vi "datascope.from_json.vi"(8 "error in":errorcluster, 10 "json":string) -> (0 "error out":errorcluster, 2 "data scope":T1)   [LabVIEW 2020, in "dataScopes.lvlib"]
uses:
  dataScopes.lvlib
  data_scope.ctl
  properties/properties.lvclass
  data_source.ctl
  type.ctl
  offset.ctl
  67163aca-3a6b-4dd5-86ca-74d13fcabb29.vi
  ab9a869c-e1cd-4f12-85c3-02f872140d20.vi
  <vilib>/JDP Science/JSONtext/Find Item.vi
  <vilib>/JDP Science/JSONtext/String Subset.vi
  <vilib>/JDP Science/JSONtext/Offset/Find Object Item Locations by Names.vi
  <vilib>/JDP Science/JSONtext/support/Quote and Escape JSON string.vi
  <vilib>/JDP Science/JSONtext/Next JSON Value.vi
  <vilib>/JDP Science/JSONtext/Parsing/Advance past whitespace.vi
  <vilib>/JDP Science/JSONtext/support/Commas Needed.vi
  <vilib>/JDP Science/JSONtext/Parsing/Advance past whitespace and comma.vi
  <vilib>/JDP Science/JSONtext/Parsing/Advance past next JSON Value (inlined COPY).vi
  <vilib>/JDP Science/JSONtext/Parsing/Advance past Item Name.vi
  <vilib>/JDP Science/JSONtext/support/quote and escape json string 2.vi
  <vilib>/JDP Science/JSONtext/Parsing/Advance past Line Ending.vi
  <vilib>/JDP Science/JSONtext/Parsing/Advance past String.vi
  <vilib>/JDP Science/JSONtext/Parsing/Advance past Number.vi
  <vilib>/JDP Science/JSONtext/Parsing/Parse Full Path or Item Name.vi
  <vilib>/JDP Science/JSONtext/Parsing/Advance past Array.vi
  <vilib>/JDP Science/JSONtext/Parsing/Advance past Object.vi
  <vilib>/JDP Science/JSONtext/support/Error Cluster From Code.vi
  <vilib>/JDP Science/JSONtext/Offset/Find Item Locations by Path.vi
  <vilib>/JDP Science/JSONtext/Parsing/Parsing Error.vi
  <vilib>/JDP Science/JSONtext/JSON text to Variant.vi
  <vilib>/JDP Science/JSONtext/LVClass Serializer/JSONtext LVClass Serializer.lvclass
  <vilib>/JDP Science/JSONtext/JSONtext.lvlib
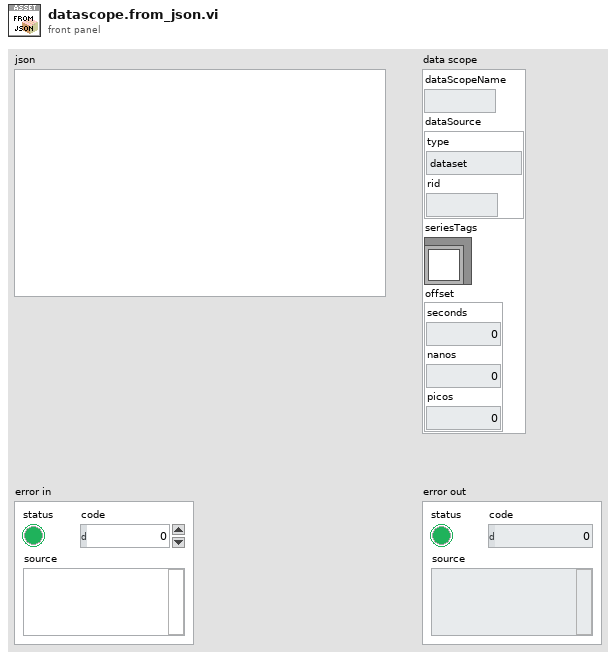
[diagram p1: front panel]
types:
  T1 = typedef "dataScopes.lvlib/data_scope.ctl" = cluster{"dataScopeName":string, "dataSource":T2, "seriesTags":refnum<class "properties.lvclass">, "offset":T4}
  T2 = typedef "dataScopes.lvlib/data_source.ctl" = cluster{"type":T3, "rid":string}
  T3 = typedef "dataScopes.lvlib/type.ctl" = enum16{"dataset", "connection", "logSet", "video"}
  T4 = typedef "dataScopes.lvlib/offset.ctl" = cluster{"seconds":i32, "nanos":i32, "picos":i32}
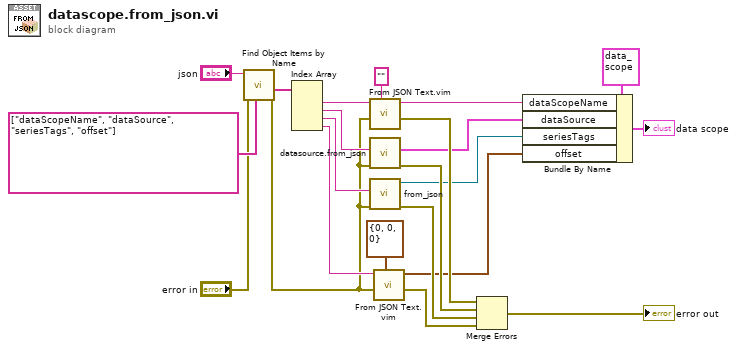
[diagram p0: block diagram]
diagram:
  n1 = call <vilib>:"Find Object Items by Name.vi"("Item Names"=string[] ["dataScopeName", "dataSource", "seriesTags", "offset"], "error in (no error)"="error in", "JSON"="json") -> ("error out"=w10:errorcluster, "<JSON>"=w20:string[])  [unwired: 6 in, 1 out]
  n2 = Index Array(array=w20) -> (element #1=w19:string, element #2=w15:string, element #3=w14:string, element #4=w12:string)  [unwired: 4 in]
  n3 = call "From JSON Text.vim"("Data Type and Default Value"="", "error in (no error)"=w10, "JSON"=w19) -> ("error out"=w9:errorcluster, "Data out"=w16:string)  [unwired: 7 in]
  n4 = call "datasource.from_json.vi"("error in"=w10, "json"=w15) -> ("error out"=w8:errorcluster, "dataSource"=w3:T2)  [unwired: 8 in]
  n5 = call "from_json.vi"("error in"=w10, "json"=w14) -> ("error out"=w7:errorcluster, "properties out"=w2:refnum<class "properties.lvclass">)  [unwired: 8 in]
  n6 = call "From JSON Text.vim"("Data Type and Default Value"=T4 {"seconds"=0, "nanos"=0, "picos"=0} ("offset"), "error in (no error)"=w10, "JSON"=w12) -> ("error out"=w6:errorcluster, "Data out"=w1:T4)  [unwired: 7 in]
  n7 = Merge Errors(w9, w8, w7, w6) -> (→"error out":errorcluster)
  n8 = Bundle By Name(cluster=T1 {"dataScopeName"="", "dataSource"={"type"=enum."dataset", "rid"=""}, "seriesTags"=refnum, "offset"={"seconds"=0, "nanos"=0, "picos"=0}} ("data scope"), "dataScopeName"=w16, "dataSource"=w3, "seriesTags"=w2, "offset"=w1) -> (→"data scope":T1)
